vi "get_phase_shift.vi"(8 "error in (no error)":errorcluster, 11 "ScanModeTS090821Circular2D in":refnum<class "ImagingModeTS090821Circular2D.lvclass">) -> (0 "error out":errorcluster, 2 "phase shift":dbl, 3 "ScanModeTS090821Circular2D out":refnum<class "ImagingModeTS090821Circular2D.lvclass">)   [LabVIEW 2010, in "ImagingModeTS090821Circular2D.lvclass"]
uses:
  ImagingModeTS090821Circular2D.lvclass
  ImagingModeTS090821Circular2D.lvclass/ImagingModeTS090821Circular2D.ctl
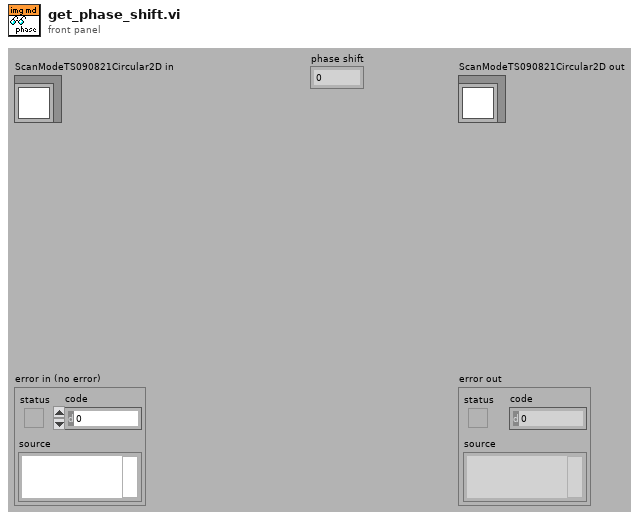
[diagram p1: front panel]
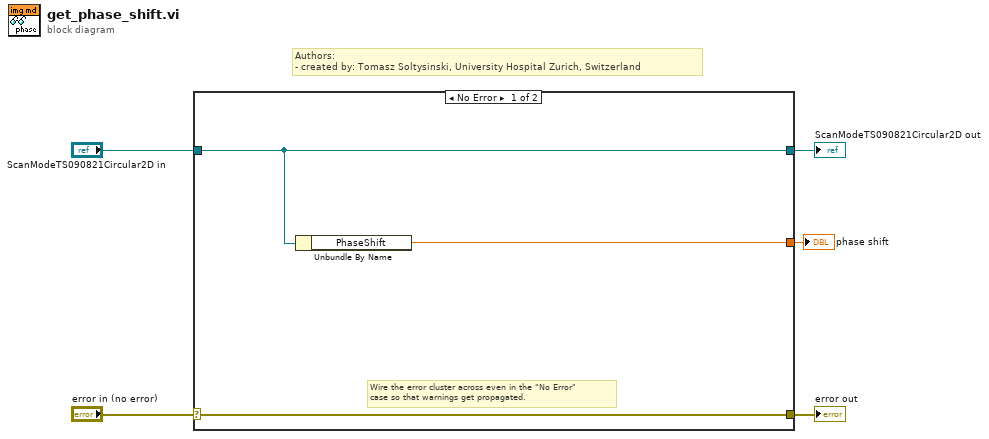
[diagram p0: block diagram]
diagram:
  # "Authors: \n- created by: Tomasz Soltysinski, University Hospital Zurich, Switzerland"
  n1 = case shown="No Error" "error in (no error)" {
    selector: "error in (no error)" -> [w8 w10]
    tunnel: [w8 w10] -> w4
    tunnel: [w7 w9] -> w2
    tunnel: "ScanModeTS090821Circular2D in" -> [w7 w9]
    tunnel: [w6 _] -> w1
    frame No Error {
      # "Wire the error cluster across even in the \"No Error\"\ncase so that warnings get propagated."
      n2 = Unbundle By Name(w7) -> ("PhaseShift"=w6:dbl)
    }
    frame Error {
    }
  }
  "error out" <- w4
  "ScanModeTS090821Circular2D out" <- w2
  "phase shift" <- w1
